vi "ReadGFGandWriteToINI.vi"(7 "remove keys":string[](array[string]), 8 "error in (no error)":errorcluster, 11 "Path":path) -> (0 "error out":errorcluster)   [LabVIEW 2012]
doc: "SciScan 1.2 160622\nThis VI reads an INI file and stores all keys in a Generalized Functional Global Variable (GFG). It then monitors updates to the GFG and writes keys back into INI file before closing. Note that the INI file only supports data type DBL or STRING. The GFG can handle any arbitrary data type, but values that are not DBL or STRING are discarded when closing and not written to INI file."
uses:
  GFG/GFGpathGet.vi
  <vilib>/Utility/config.llb/Write Key (Double).vi
  <vilib>/Utility/config.llb/Write Key (String).vi
  <vilib>/Utility/config.llb/Write Key (Boolean).vi
  <vilib>/Utility/config.llb/NI_LVConfig.lvlib
  GFG/GFG library.lvlib
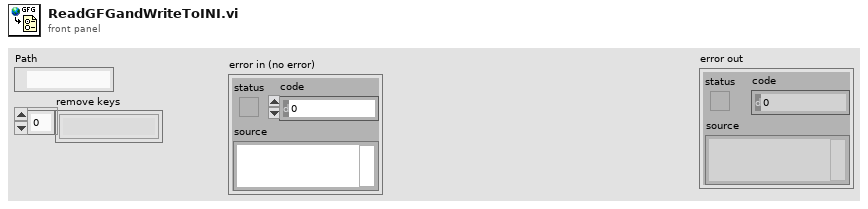
[diagram p1: front panel]
types:
  T1 = typedef "NI_LVConfig.lvlib/Config Data RefNum.ctl" = refnum<k1>
  T2 = typedef "VariantType.lvlib/Type.ctl" = enum8{"Invalid Type", "Void", "I8", "I16", "I32", "I64", "U8", "U16", "U32", "U64", "Single Float", "Double Float", "Extended Float", "Single Complex", "Double Complex", "Extended Complex", "Enum U8", "Enum U16", "Enum U32", "Enum U64", "Single Float With Unit", "Double Float With Unit", "Extended Float With Unit", "Single Complex with Unit", "Double Complex with Unit", "Extended Complex with Unit", "Boolean", "String", "Path", "Picture", "Tag", "Array", "Cluster", "Variant", "LV Variant", "Waveform", "Timestamp", "Digital Waveform", "Digital Data", "ExpressData", "Refnum", "External Data", "VI", "Poly VI", "LabVIEW Class Instance", "Fixed Point"}
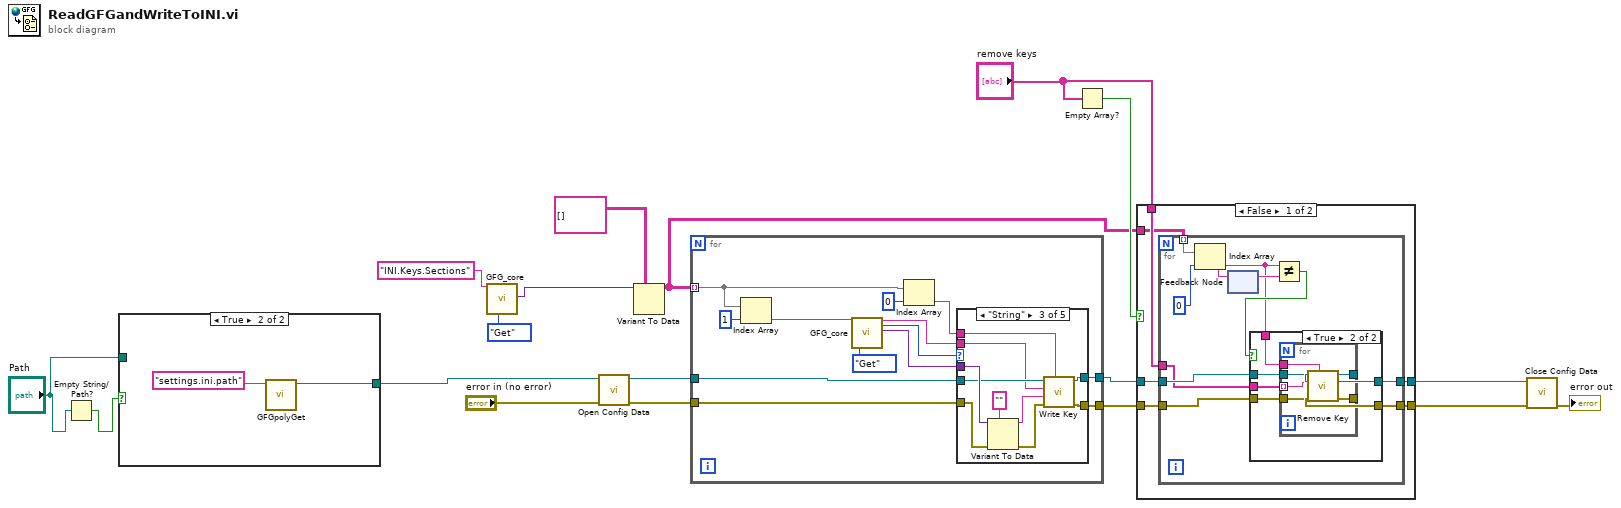
[diagram p0: block diagram]
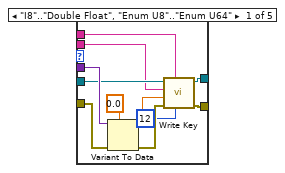
[diagram p5: hidden frame]
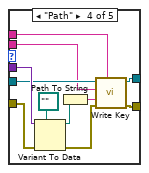
[diagram p7: hidden frame]
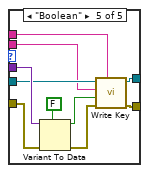
[diagram p8: hidden frame]
diagram:
  n1 = Empty String/Path?(string/path="Path") -> (empty?=w8:bool)
  n2 = case shown="True" w8 {
    tunnel: [w19 w20] -> w10
    tunnel: "Path" -> [w19 _]
    frame False {
    }
    frame True {
      n3 = call-poly "GFGpolyGet.vi"("Variable Name in"="settings.ini.path") -> ("Path"=w20:path)  [unwired: 8 in, 2 out]
    }
  }
  n4 = call "GFG_core.vi"("Variable Name in"="INI.Keys.Sections", "Action"=enum16{"Init", "Set", "Get"}."Get") -> ("Variant Out"=w15:variant)  [unwired: 11 in, 6 out]
  n5 = call <vilib>:"Open Config Data.vi"("error in (no error)"="error in (no error)", "configuration file path"=w10) -> ("error out"=w12:errorcluster, "refnum"=w13:T1)  [unwired: 7 in, 1 out]
  n6 = Variant To Data(type=string[][] [], Variant=w15) -> (data=w1:string[][])  [unwired: 1 in, 1 out]
  n7 = for {
    tunnel: w1 -> [w32] mode=indexing
    tunnel: [w26] -> w7
    tunnel: w13 -> [w25]
    tunnel: w12 -> [w27]
    tunnel: [w24] -> w5
    n8 = Index Array(array=w32, index=1) -> (element=w30:string)
    n9 = call "GFG_core.vi"("Variable Name in"=w30, "Action"=enum16{"Init", "Set", "Get"}."Get") -> ("Variable Name Out"=w23:string, "Data Type Out"=w29:T2, "Variant Out"=w28:variant)  [unwired: 11 in, 4 out]
    n10 = Index Array(array=w32, index=0) -> (element=w22:string)
    n11 = case shown="\"String\"" w29 {
      tunnel: w28 -> [w44 _ w57 w68 w78]
      tunnel: [w41 w47 w54 w66 w75] -> w26
      tunnel: w27 -> [w40 w47 w53 w65 w74]
      tunnel: w25 -> [w39 w46 w52 w64 w73]
      tunnel: [w38 w46 w51 w63 w72] -> w24
      tunnel: w23 -> [w37 _ w50 w62 w71]
      tunnel: w22 -> [w36 _ w49 w61 w70]
      frame "I8".."Double Float", "Enum U8".."Enum U64" {
        n12 = Variant To Data(error in=w40, type=0.0, Variant=w44) -> (data=w43:dbl, error out=w42:errorcluster)
        n13 = call-poly <vilib>:"Write Key.vi"("precision (6)"=i16 12, "section"=w36, "error in (no error)"=w42, "value"=w43, "key"=w37, "refnum"=w39) -> ("error out"=w41:errorcluster, "refnum out"=w38:T1)  [unwired: 3 in, 1 out]
      }
      frame Default {
      }
      frame "String" {
        n14 = Variant To Data(error in=w53, type="" ("Variable Name Out"), Variant=w57) -> (data=w56:string, error out=w55:errorcluster)
        n15 = call-poly <vilib>:"Write Key.vi"("section"=w49, "error in (no error)"=w55, "value"=w56, "key"=w50, "refnum"=w52) -> ("error out"=w54:errorcluster, "refnum out"=w51:T1)  [unwired: 4 in, 1 out]
      }
      frame "Path" {
        n16 = Variant To Data(error in=w65, type=path "" ("configuration file path 2"), Variant=w68) -> (data=w58:path, error out=w67:errorcluster)
        n17 = Path To String(path=w58) -> (string=w59:string)
        n18 = call-poly <vilib>:"Write Key.vi"("section"=w61, "error in (no error)"=w67, "value"=w59, "key"=w62, "refnum"=w64) -> ("error out"=w66:errorcluster, "refnum out"=w63:T1)  [unwired: 4 in, 1 out]
      }
      frame "Boolean" {
        n19 = Variant To Data(error in=w74, type=FALSE, Variant=w78) -> (data=w77:bool, error out=w76:errorcluster)
        n20 = call-poly <vilib>:"Write Key.vi"("section"=w70, "error in (no error)"=w76, "value"=w77, "key"=w71, "refnum"=w73) -> ("error out"=w75:errorcluster, "refnum out"=w72:T1)  [unwired: 4 in, 1 out]
      }
    }
  }
  n21 = Empty Array?(array="remove keys") -> (empty?=w3:bool)
  n22 = case shown="False" w3 {
    tunnel: w7 -> [w84 w109]
    tunnel: [w83 w109] -> w6
    tunnel: w5 -> [w82 w110]
    tunnel: [w81 w110] -> w4
    tunnel: "remove keys" -> [w80 _]
    tunnel: w1 -> [w79 _]
    frame False {
      n23 = for {
        tunnel: w84 -> [w94]
        tunnel: [w93] -> w83
        tunnel: w82 -> [w92]
        tunnel: [w91] -> w81
        tunnel: w80 -> [w90]
        tunnel: w79 -> [w88] mode=indexing
        n24 = Index Array(array=w88, index=0) -> (element=w85:string)
        n25 = feedback-in #1(w85) -> ()
        n26 = feedback #1() -> (w87:string)  [unwired: 1 in]
        n27 = Not Equal?(x=w85, y=w87) -> (x != y?=w86:bool)
        n28 = case shown="True" w86 {
          tunnel: w94 -> [w95 w102]
          tunnel: [w95 w101] -> w93
          tunnel: w92 -> [w96 w100]
          tunnel: [w96 w99] -> w91
          tunnel: w90 -> [_ w98]
          tunnel: w85 -> [_ w97]
          frame False {
          }
          frame True {
            n29 = for {
              tunnel: w102 -> [w108]
              tunnel: [w107] -> w101
              tunnel: w100 -> [w106]
              tunnel: [w105] -> w99
              tunnel: w98 -> [w104] mode=indexing
              tunnel: w97 -> [w103]
              n30 = call <vilib>:"Remove Key.vi"("section"=w103, "error in (no error)"=w108, "key"=w104, "refnum"=w106) -> ("error out"=w107:errorcluster, "refnum out"=w105:T1)  [unwired: 5 in, 1 out]
            }
          }
        }
      }
    }
    frame True {
    }
  }
  n31 = call <vilib>:"Close Config Data.vi"("error in (no error)"=w6, "refnum"=w4) -> ("error out"=→"error out":errorcluster)  [unwired: 8 in, 1 out]
